vi "Read Offset.vi"(8 "error in":errorcluster, 10 "Offset":T1, 11 "Config Manager in":refnum<class "Config Manager Class.lvclass">) -> (0 "error out":errorcluster, 2 "Vec3d out":refnum<class "Vec3d Class.lvclass">, 3 "Config Manager out":refnum<class "Config Manager Class.lvclass">)   [LabVIEW 2011, in "Config Manager Class.lvclass"]
uses:
  Config Manager Class.lvclass
  Vec3d Class/Vec3d Class.lvclass
  Type Definitions/Offset.ctl
  Config Manager Class.lvclass/Config Manager Class.ctl
  <vilib>/Utility/config.llb/Read Key (String).vi
  <vilib>/Utility/config.llb/NI_LVConfig.lvlib
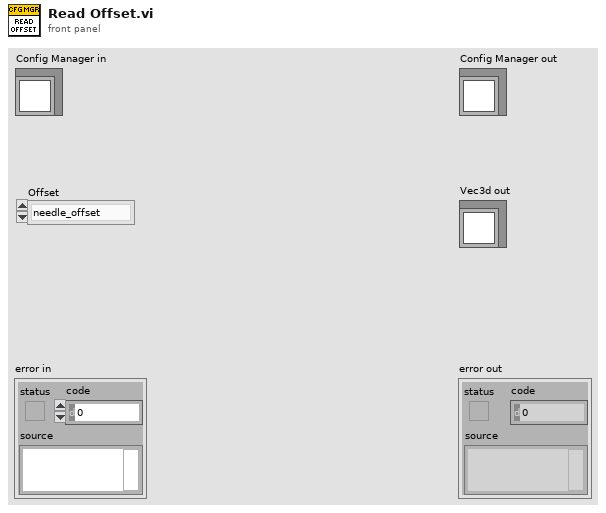
[diagram p1: front panel]
types:
  T1 = typedef "Offset.ctl" = enum16{"needle_offset", "tool_holder_offset"}
  T2 = typedef "NI_LVConfig.lvlib/Config Data RefNum.ctl" = refnum<k1>
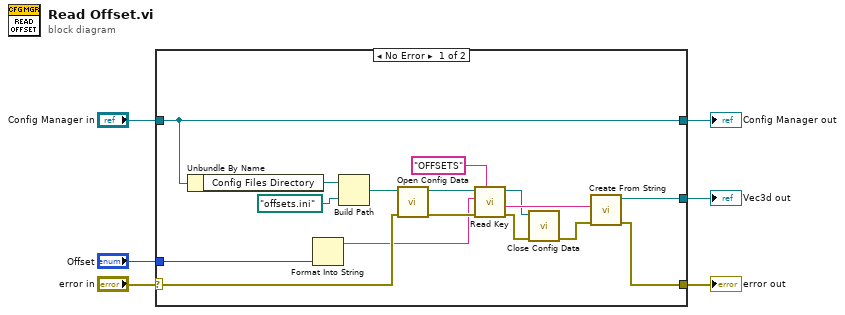
[diagram p0: block diagram]
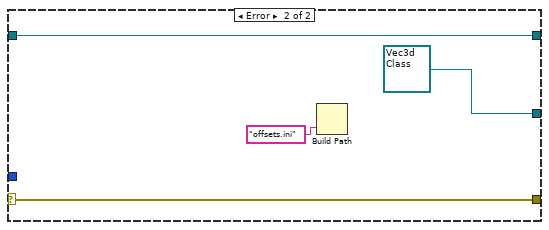
[diagram p2: hidden frame]
diagram:
  n1 = case shown="No Error" "error in" {
    selector: "error in" -> [w18 w26]
    tunnel: [w13 w26] -> w5
    tunnel: [w16 refnum<class "Vec3d Class.lvclass"> refnum ("Vec3d out")] -> w6
    tunnel: "Offset" -> [w12 _]
    tunnel: "Config Manager in" -> [w10 w23]
    tunnel: [w10 w23] -> w2
    frame No Error {
      n2 = Unbundle By Name(w10) -> ("Config Files Directory"=w9:path)
      n3 = Format Into String(w12) -> (resulting string=w11:string)  [unwired: 3 in, 1 out]
      n4 = Build Path(base path=w9, name or relative path=path "offsets.ini") -> (appended path=w7:path)
      n5 = call <vilib>:"Open Config Data.vi"("error in (no error)"=w18, "configuration file path"=w7) -> ("error out"=w20:errorcluster, "refnum"=w22:T2)  [unwired: 7 in, 1 out]
      n6 = call-poly <vilib>:"Read Key.vi"("section"="OFFSETS", "error in (no error)"=w20, "key"=w11, "refnum"=w22) -> ("error out"=w15:errorcluster, "value"=w21:string, "refnum out"=w17:T2)  [unwired: 4 in, 1 out]
      n7 = call <vilib>:"Close Config Data.vi"("error in (no error)"=w15, "refnum"=w17) -> ("error out"=w14:errorcluster)  [unwired: 8 in, 1 out]
      n8 = call "Create From String.vi"("error in"=w14, "Input String"=w21) -> ("error out"=w13:errorcluster, "Vec3d out"=w16:refnum<class "Vec3d Class.lvclass">)  [unwired: 8 in]
    }
    frame Error {
      n9 = Build Path(name or relative path="offsets.ini") -> ()  [unwired: 1 in, 1 out]
    }
  }
  "error out" <- w5
  "Config Manager out" <- w2
  "Vec3d out" <- w6
